vi "KepcoDCPwr Configure Current Mode.vi"(0 "VISA Session":refnum<visa-resource-name>, 1 "Transient Time (0.0005 seconds)":dbl=0.0005 format="%^.2e", 5 "Model In":string, 7 "Channel Name (\"\")":string, 9 "Mode (Fixed)":T1(ring), 11 "error in (no error)":errorcluster {"code" format="%.0x"}) -> (4 "VISA Session Out":refnum<visa-resource-name>, 6 "Model Out":string, 8 "channel name out (\"\")":string="\"\"" caption="channel name Out (\"\")", 15 "error out":errorcluster {"code" format="%.0x"})   [LabVIEW 2020]
doc: "This VI configures the current mode.\n\nNote:\n\nThis VI is available only for instruments with interface card BIT 4886."
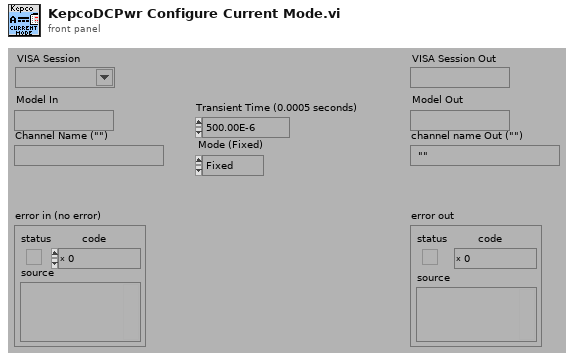
[diagram p1: front panel]
types:
  T1 = enum16{"Fixed", "List", "Transient", "External", "Gain", "Protect", "Additive"}
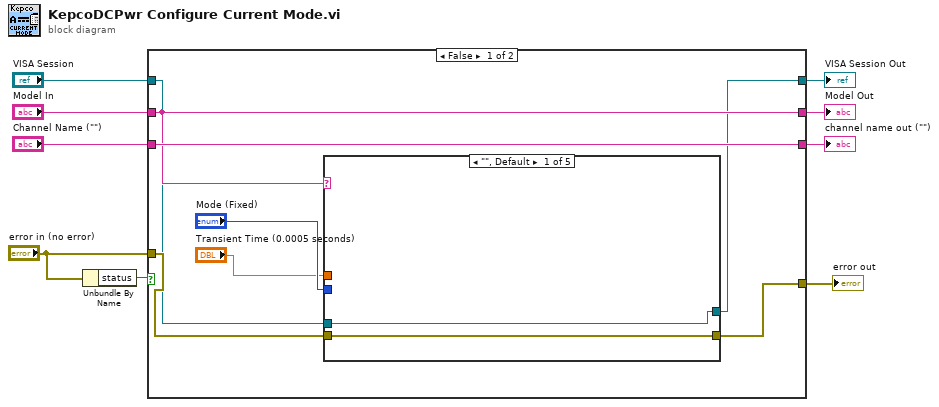
[diagram p0: block diagram]
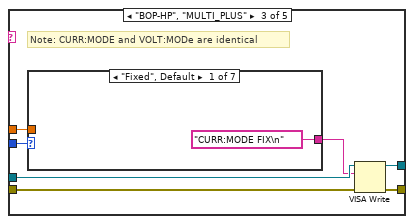
[diagram p3: hidden frame]
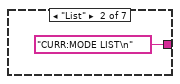
[diagram p4: hidden frame]
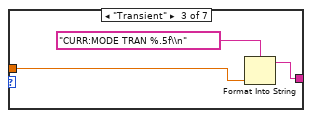
[diagram p5: hidden frame]
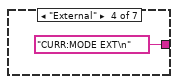
[diagram p6: hidden frame]
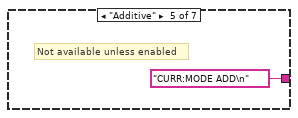
[diagram p7: hidden frame]
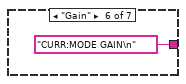
[diagram p8: hidden frame]
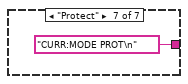
[diagram p9: hidden frame]
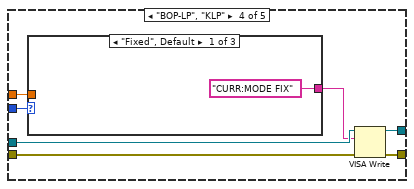
[diagram p10: hidden frame]
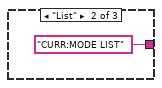
[diagram p11: hidden frame]
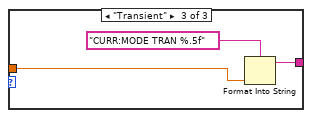
[diagram p12: hidden frame]
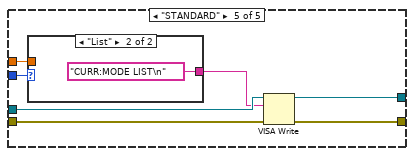
[diagram p13: hidden frame]
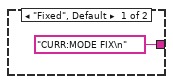
[diagram p14: hidden frame]
diagram:
  n1 = Unbundle By Name("error in (no error)") -> ("status"=w5:bool)
  n2 = case shown="False" w5 {
    tunnel: [w15 w61] -> w9
    tunnel: "VISA Session" -> [w12 w62]
    tunnel: [w11 w62] -> w7
    tunnel: "error in (no error)" -> [w16 w61]
    tunnel: "Model In" -> [w14 w60]
    tunnel: "Channel Name (\"\")" -> [w17 w59]
    tunnel: [w14 w60] -> w2
    tunnel: [w17 w59] -> w1
    frame False {
      n3 = case shown="\"\", Default" w14 {
        tunnel: w16 -> [w19 w20 w28 w44 w56]
        tunnel: [w19 w20 w27 w43 w55] -> w15
        tunnel: w12 -> [w18 w21 w26 w42 w54]
        tunnel: [w18 w21 w25 w41 w53] -> w11
        tunnel: "Transient Time (0.0005 seconds)" -> [_ _ w24 w40 w52]
        tunnel: "Mode (Fixed)" -> [_ _ w22 w38 w50]
        frame "", Default {
        }
        frame "MULTI" {
        }
        frame "BOP-HP", "MULTI_PLUS" {
          # "Note: CURR:MODE and VOLT:MODe are identical"
          n4 = case shown="\"Fixed\", Default" w22 {
            tunnel: w24 -> [_ _ w32 _ _ _ _]
            tunnel: ["CURR:MODE FIX\n" "CURR:MODE LIST\n" w31 "CURR:MODE EXT\n" "CURR:MODE ADD\n" "CURR:MODE GAIN\n" "CURR:MODE PROT\n"] -> w23
            frame "Fixed", Default {
            }
            frame "List" {
            }
            frame "Transient" {
              n5 = Format Into String(format string="CURR:MODE TRAN %.5f\\n", w32) -> (resulting string=w31:string)  [unwired: 2 in, 1 out]
            }
            frame "External" {
            }
            frame "Additive" {
              # "Not available unless enabled"
            }
            frame "Gain" {
            }
            frame "Protect" {
            }
          }
          n6 = VISA Write(VISA resource name=w26, write buffer=w23, error in (no error)=w28) -> (VISA resource name out=w25:refnum<visa-resource-name>, error out=w27:errorcluster)  [unwired: 1 out]
        }
        frame "BOP-LP", "KLP" {
          n7 = case shown="\"Fixed\", Default" w38 {
            tunnel: w40 -> [_ _ w48]
            tunnel: ["CURR:MODE FIX" "CURR:MODE LIST" w47] -> w39
            frame "Fixed", Default {
            }
            frame "List" {
            }
            frame "Transient" {
              n8 = Format Into String(format string="CURR:MODE TRAN %.5f", w48) -> (resulting string=w47:string)  [unwired: 2 in, 1 out]
            }
          }
          n9 = VISA Write(VISA resource name=w42, write buffer=w39, error in (no error)=w44) -> (VISA resource name out=w41:refnum<visa-resource-name>, error out=w43:errorcluster)  [unwired: 1 out]
        }
        frame "STANDARD" {
          n10 = case shown="\"List\"" w50 {
            tunnel: w52 -> [_ _]
            tunnel: ["CURR:MODE FIX\n" "CURR:MODE LIST\n"] -> w51
            frame "Fixed", Default {
            }
            frame "List" {
            }
          }
          n11 = VISA Write(VISA resource name=w54, write buffer=w51, error in (no error)=w56) -> (VISA resource name out=w53:refnum<visa-resource-name>, error out=w55:errorcluster)  [unwired: 1 out]
        }
      }
    }
    frame True {
    }
  }
  "error out" <- w9
  "VISA Session Out" <- w7
  "channel name out (\"\")" <- w1
  "Model Out" <- w2
